vi "Waka battery update.vi"(8 "error in (no error)":errorcluster, 9 "Supply Voltage":dbl, 10 "Supply Current":dbl, 11 "Frame Signal Conversion in":refnum<class "Frame Signal Conversion.lvclass">) -> (0 "error out":errorcluster)   [LabVIEW 2024]
uses:
  PROD_LabView_Libraries/PCAN-XNET/Frame signal conversion/Frame Signal Conversion Version 8/Frame Signal Conversion.lvclass
  PROD_LabView_Libraries/PCAN-XNET/BCI Signal cluster.ctl
  <instrlib>/KDI Digital Instrumentation/API_for_PCAN_BASIC_FD/TPCANHandle.ctl
  PROD_LabView_Libraries/PCAN-XNET/PCan_Xnet.lvlib
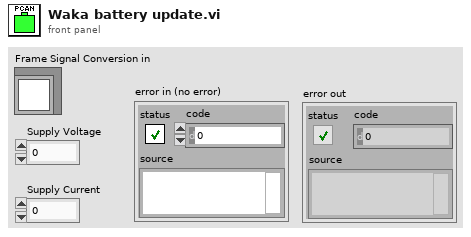
[diagram p1: front panel]
types:
  T1 = typedef "PCan_Xnet.lvlib/BCI Signal cluster.ctl" = cluster{"BAT_CURRENT_PDO":dbl, "BAT_BALANCING_PDO":bool, "BAT_CHARGING_PDO":bool, "BAT_DISCHARGING_PDO":bool, "BAT_EOC_PDO":bool, "BAT_HEARTBEAT":i8, "BAT_LASTWARNING_PDO":u16, "BAT_MEASCAP":u16, "BAT_REQCHGCURR_PDO":dbl, "BAT_REQCHGVOLT_PDO":dbl, "BAT_SOC_PDO":u8, "BAT_SOH_PDO":u8, "BAT_STATE_PDO":bool, "BAT_VOLTS_PDO":dbl, "BAT_WARNING_PDO":u16, "BAT_LASTERROR_PDO":u16, "BAT_REMAININGCAP_PDO":u16, "BAT_TEMP_PDO":i16}
  T2 = typedef "TPCANHandle.ctl" = enum16{"PCAN_NONEBUS  0x000", "PCAN_ISABUS1  0x21", "PCAN_ISABUS2  0x22", "PCAN_ISABUS3  0x23", "PCAN_ISABUS4  0x24", "PCAN_ISABUS5  0x25", "PCAN_ISABUS6  0x26", "PCAN_ISABUS7  0x27", "PCAN_ISABUS8  0x28", "PCAN_DNGBUS1  0x31", "PCAN_PCIBUS1  0x41", "PCAN_PCIBUS1  0x42", "PCAN_PCIBUS1  0x43", "PCAN_PCIBUS1  0x44", "PCAN_PCIBUS1  0x45", "PCAN_PCIBUS1  0x46", "PCAN_PCIBUS1  0x47", "PCAN_PCIBUS1  0x48", "PCAN_PCIBUS1  0x409", "PCAN_PCIBUS1  0x40A", "PCAN_PCIBUS1  0x40B", "PCAN_PCIBUS1  0x40C", "PCAN_PCIBUS1  0x40D", "PCAN_PCIBUS1  0x40E", "PCAN_PCIBUS1  0x40F", "PCAN_PCIBUS1  0x410", "PCAN_USBBUS1  0x51", "PCAN_USBBUS2  0x52", "PCAN_USBBUS3  0x53", "PCAN_USBBUS4  0x54", "PCAN_USBBUS5  0x55", "PCAN_USBBUS6  0x56", "PCAN_USBBUS7  0x57", "PCAN_USBBUS8  0x58", "PCAN_USBBUS9  0x509", "PCAN_USBBUS10  0x50A", "PCAN_USBBUS11  0x50B", "PCAN_USBBUS12  0x50C", "PCAN_USBBUS13  0x50D", "PCAN_USBBUS14  0x50E", "PCAN_USBBUS15  0x50F", "PCAN_USBBUS16  0x510", "PCAN_PCCBUS1  0x61", "PCAN_PCCBUS2  0x62", "PCAN_LANBUS1  0x801", "PCAN_LANBUS2  0x802", "PCAN_LANBUS3  0x803", "PCAN_LANBUS4  0x804", "PCAN_LANBUS5  0x805", "PCAN_LANBUS6  0x806", "PCAN_LANBUS7  0x807", "PCAN_LANBUS8  0x808", "PCAN_LANBUS9  0x809", "PCAN_LANBUS10  0x80A", "PCAN_LANBUS11  0x80B", "PCAN_LANBUS12  0x80C", "PCAN_LANBUS13  0x80D", "PCAN_LANBUS14  0x80E", "PCAN_LANBUS15  0x80F", "PCAN_LANBUS16  0x810"}
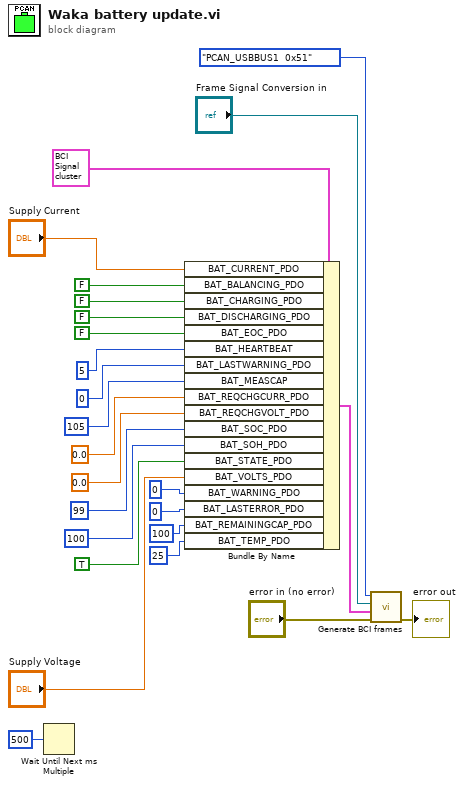
[diagram p0: block diagram]
diagram:
  n1 = Wait Until Next ms Multiple(millisecond multiple=u32 500) -> ()  [unwired: 1 out]
  n2 = Bundle By Name(cluster=T1 {"BAT_CURRENT_PDO"=0.0, "BAT_BALANCING_PDO"=FALSE, "BAT_CHARGING_PDO"=FALSE, "BAT_DISCHARGING_PDO"=FALSE, "BAT_EOC_PDO"=FALSE, "BAT_HEARTBEAT"=5, "BAT_LASTWARNING_PDO"=0, "BAT_MEASCAP"=105, "BAT_REQCHGCURR_PDO"=0.0, "BAT_REQCHGVOLT_PDO"=0.0, "BAT_SOC_PDO"=0, "BAT_SOH_PDO"=100, "BAT_STATE_PDO"=FALSE, "BAT_VOLTS_PDO"=5.0, "BAT_WARNING_PDO"=0, "BAT_LASTERROR_PDO"=0, "BAT_REMAININGCAP_PDO"=105, "BAT_TEMP_PDO"=25} ("Battery signals to send"), "BAT_CURRENT_PDO"="Supply Current", "BAT_BALANCING_PDO"=FALSE, "BAT_CHARGING_PDO"=FALSE, "BAT_DISCHARGING_PDO"=FALSE, "BAT_EOC_PDO"=FALSE, "BAT_HEARTBEAT"=i8 5, "BAT_LASTWARNING_PDO"=u16 0, "BAT_MEASCAP"=u16 105, "BAT_REQCHGCURR_PDO"=0.0, "BAT_REQCHGVOLT_PDO"=0.0, "BAT_SOC_PDO"=u8 99, "BAT_SOH_PDO"=u8 100, "BAT_STATE_PDO"=TRUE, "BAT_VOLTS_PDO"="Supply Voltage", "BAT_WARNING_PDO"=u16 0, "BAT_LASTERROR_PDO"=u16 0, "BAT_REMAININGCAP_PDO"=u16 100, "BAT_TEMP_PDO"=i16 25) -> (w4:T1)
  n3 = call "Generate BCI frames.vi"("error in (no error)"="error in (no error)", "Battery signals to send"=w4, "Frame Signal Conversion"="Frame Signal Conversion in", "TPCANHandle"=TPCANHandle."PCAN_USBBUS1  0x51") -> ("error out"=→"error out":errorcluster)  [unwired: 5 in, 2 out]
